vi "Handling AI param_Dll.vi"(4 "APCcode":i32[](array[numeric]), 5 "initialise":bool, 6 "AP":dbl[](array[numeric]), 7 "connect":bool[](array[boolean]), 8 "error in":errorcluster, 9 "input registers":u16[][](array[numeric]) format="%x", 10 "AI.AIP":refnum<data-value>, 11 "AI in":T1) -> (0 "error":errorcluster, 3 "AI out":T1)   [LabVIEW 2019, in "Inputs.lvlib"]
uses:
  Inputs.lvlib
  Ctl/AI short.ctl
  Ctl/Parameter State.ctl
  Timer Delay/Timers.lvlib
  src/libInputs.dll
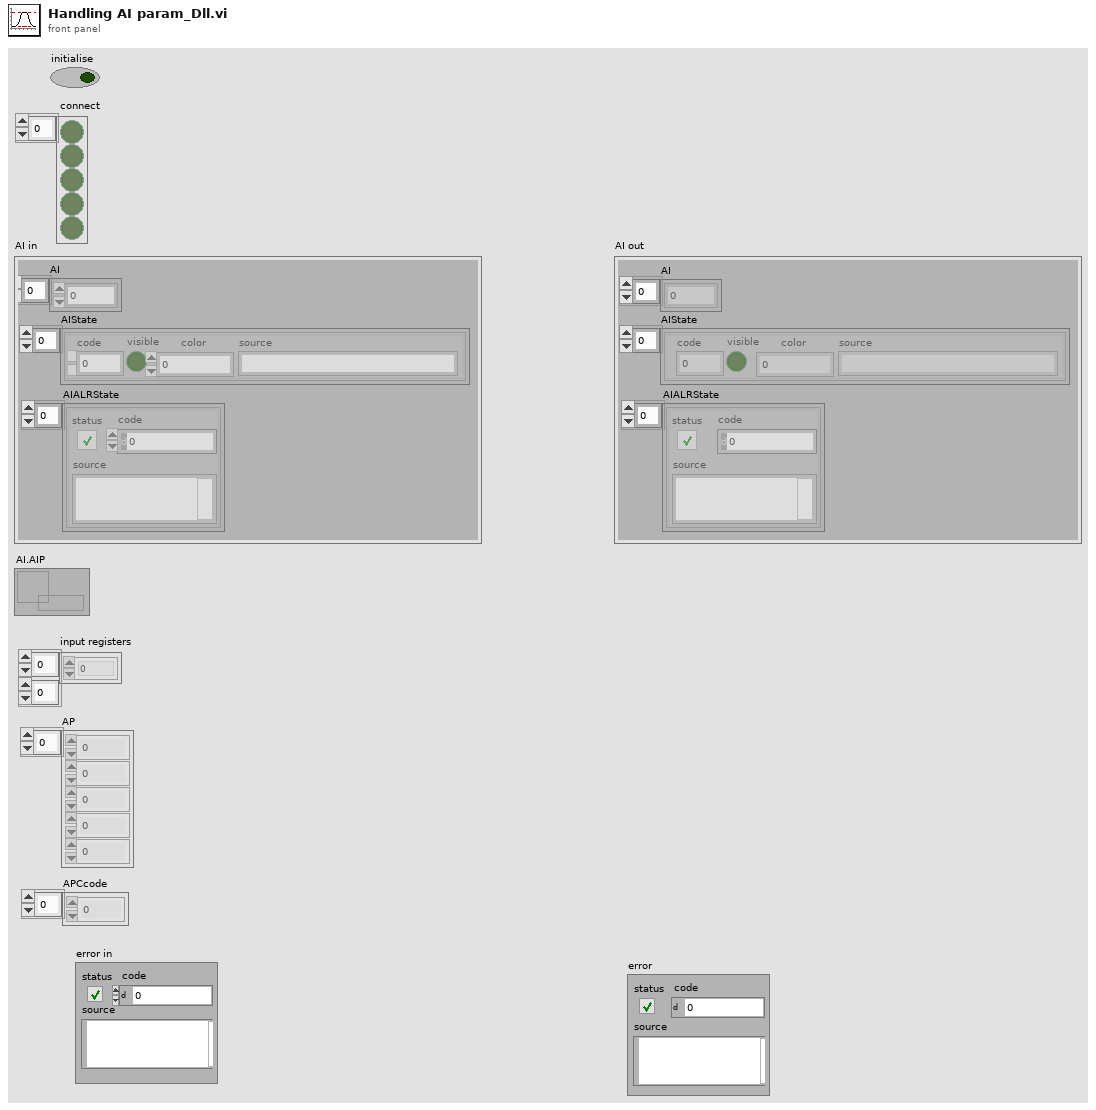
[diagram p1: front panel]
types:
  T1 = typedef "Inputs.lvlib/AI short.ctl" = cluster{"AI":dbl[], "AIState":T2[], "AIALRState":errorcluster[]}
  T2 = typedef "Inputs.lvlib/Parameter State.ctl" = cluster{"code":i32, "visible":bool, "color":u32, "source":string}
  T3 = cluster{"source":string, "color":u32, "visible":bool}[]
  T4 = cluster{"Filter PV_OUT":dbl, "Filter T":dbl, "Filter dT":dbl, "RS32 Q":u64}[]
  T5 = cluster{"Filter PV_OUT":dbl, "Filter T":dbl, "Filter dT":dbl, "RS32 Q":u64}
  T6 = cluster{"source":string, "color":u32, "visible":bool}
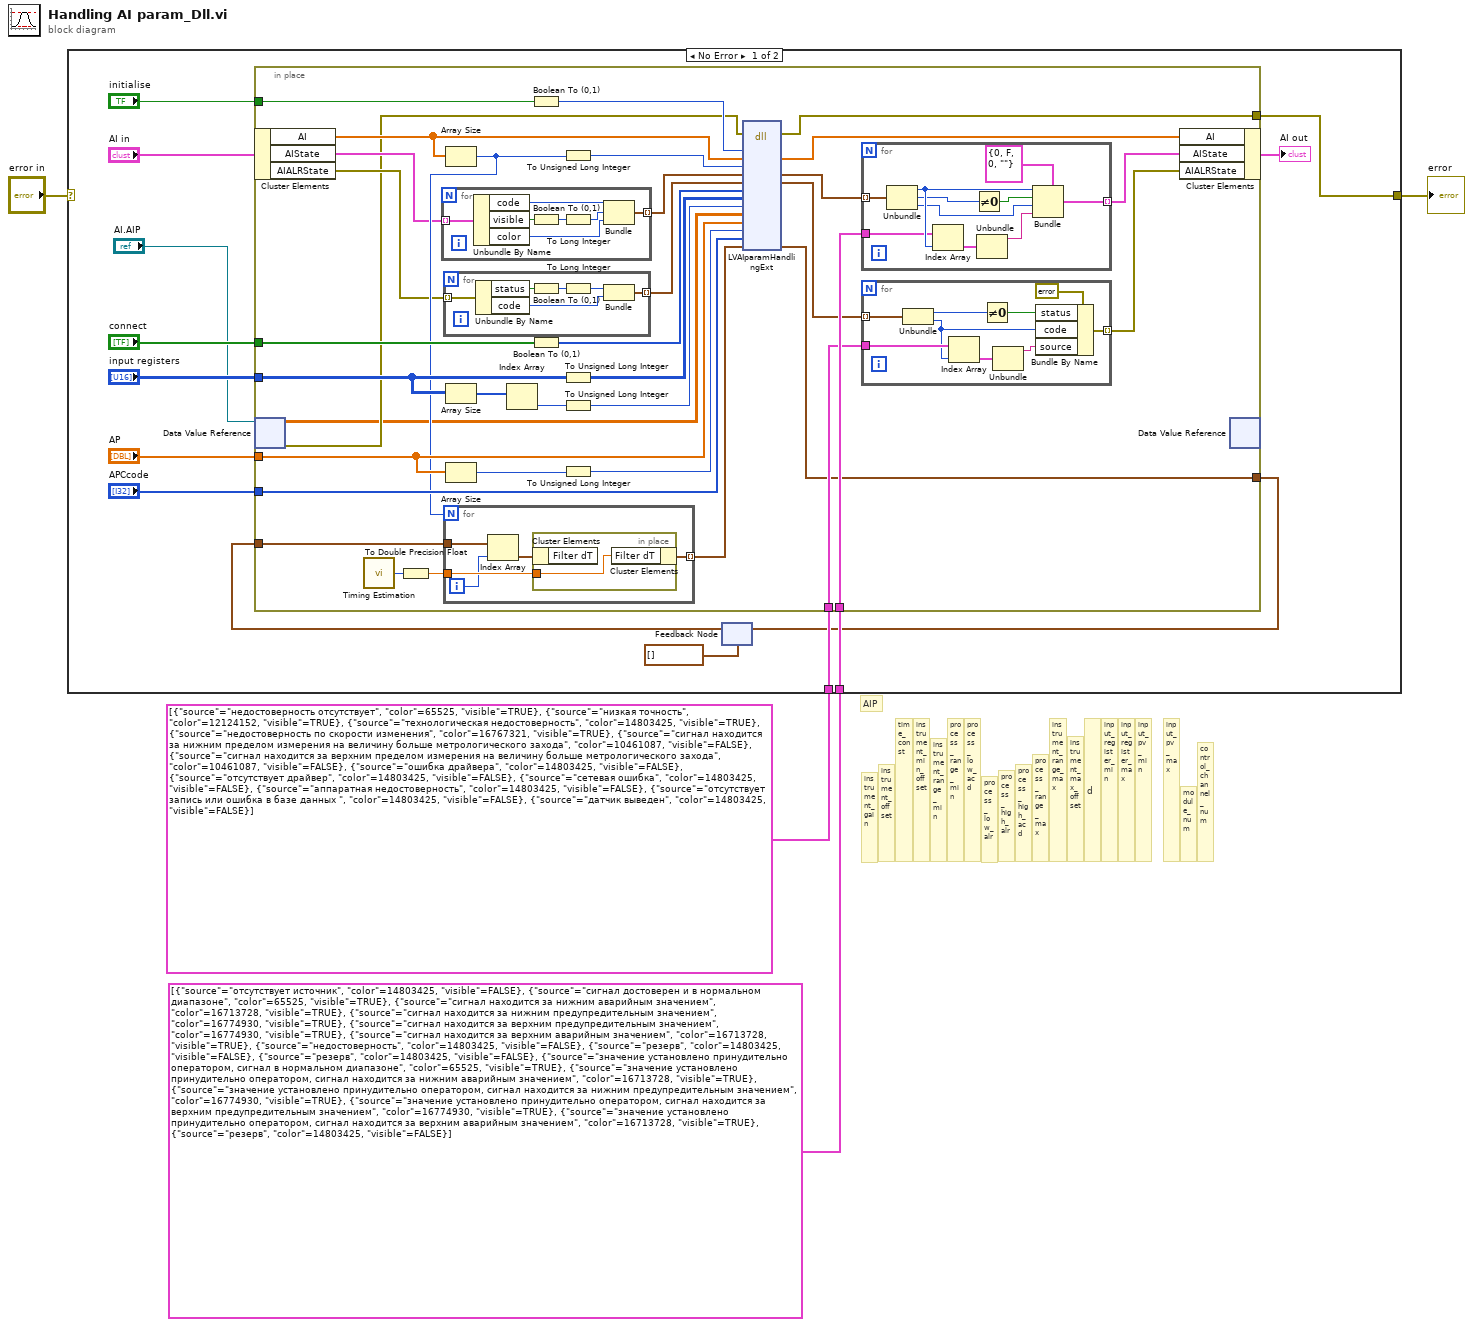
[diagram p0: block diagram]
diagram:
  # "AIP"
  # "control_channel_num"
  # "module_num"
  # "input_pv_max"
  # "input_pv_min"
  # "input_register_max"
  # "input_register_min"
  # "d"
  # "instrument_max_offset"
  # "instrument_range_max"
  # "process_range_max"
  # "process_high_acd"
  # "process_high_alr"
  # "process_low_alr"
  # "process_low_acd"
  # "process_range_min"
  # "instrument_range_min"
  # "instrument_min_offset"
  # "time_const"
  # "instrument_gain"
  # "instrument_offset"
  n1 = case shown="No Error" "error in" {
    selector: "error in" -> [_ w92]
    tunnel: T3 [{"source"="отсутствует источник", "color"=14803425, "visible"=FALSE}, {"source"="сигнал достоверен и в нормальном диапазоне", "color"=65525, "visible"=TRUE}, {"source"="сигнал находится за нижним аварийным значением", "color"=16713728, "visible"=TRUE}, {"source"="сигнал находится за нижним предупредительным значением", "color"=16774930, "visible"=TRUE}, {"source"="сигнал находится за верхним предупредительным значением", "color"=16774930, "visible"=TRUE}, {"source"="сигнал находится за верхним аварийным значением", "color"=16713728, "visible"=TRUE}, {"source"="недостоверность", "color"=14803425, "visible"=FALSE}, {"source"="резерв", "color"=14803425, "visible"=FALSE}, {"source"="резерв", "color"=14803425, "visible"=FALSE}, {"source"="значение установлено принудительно оператором, сигнал в нормальном диапазоне", "color"=65525, "visible"=TRUE}, {"source"="значение установлено принудительно оператором, сигнал находится за нижним аварийным значением", "color"=16713728, "visible"=TRUE}, {"source"="значение установлено принудительно оператором, сигнал находится за нижним предупредительным значением", "color"=16774930, "visible"=TRUE}, {"source"="значение установлено принудительно оператором, сигнал находится за верхним предупредительным значением", "color"=16774930, "visible"=TRUE}, {"source"="значение установлено принудительно оператором, сигнал находится за верхним аварийным значением", "color"=16713728, "visible"=TRUE}, {"source"="резерв", "color"=14803425, "visible"=FALSE}] -> [w16 _]
    tunnel: T3 [{"source"="недостоверность отсутствует", "color"=65525, "visible"=TRUE}, {"source"="низкая точность", "color"=12124152, "visible"=TRUE}, {"source"="технологическая недостоверность", "color"=14803425, "visible"=TRUE}, {"source"="недостоверность по скорости изменения", "color"=16767321, "visible"=TRUE}, {"source"="сигнал находится за нижним пределом измерения на величину больше метрологического захода", "color"=10461087, "visible"=FALSE}, {"source"="сигнал находится за верхним пределом измерения на величину больше метрологического захода", "color"=10461087, "visible"=FALSE}, {"source"="ошибка драйвера", "color"=14803425, "visible"=FALSE}, {"source"="отсутствует драйвер", "color"=14803425, "visible"=FALSE}, {"source"="сетевая ошибка", "color"=14803425, "visible"=FALSE}, {"source"="аппаратная недостоверность", "color"=14803425, "visible"=FALSE}, {"source"="отсутствует запись или ошибка в базе данных ", "color"=14803425, "visible"=FALSE}, {"source"="датчик выведен", "color"=14803425, "visible"=FALSE}] -> [w15 _]
    tunnel: [w8 w92] -> w2
    frame No Error {
      n2 = feedback #1(T4 []) -> (w10:T4)
      n3 = in-place {
        in-place-border: "initialise" -> [w53]
        in-place-border: "connect" -> [w52]
        in-place-border: w16 -> [w51]
        in-place-border: w15 -> [w50]
        in-place-border: "APCcode" -> [w49]
        in-place-border: "AP" -> [w48]
        in-place-border: "input registers" -> [w47]
        in-place-border: [w44] -> w11
        in-place-border: w10 -> [w43]
        in-place-border: [w27] -> w8
        n4 = in-place-cluster #2("AI in") -> ("AI"=w26:dbl[], "AIState"=w25:T2[], "AIALRState"=w24:errorcluster[])
        n5 = in-place-dvr #3("AI.AIP") -> (w19:dbl[][], w20:errorcluster)
        n6 = call "Timing Estimation.vi"() -> ("dt (ms) out"=w46:u32)  [unwired: 9 in]
        n7 = To Double Precision Float(number=w46) -> (double precision float=w45:dbl)
        n8 = for {
          tunnel: w25 -> [w66] mode=indexing
          tunnel: [w65] -> w37 mode=indexing
          n9 = Unbundle By Name(w66) -> ("code"=w64:i32, "visible"=w62:bool, "color"=w63:u32)
          n10 = Boolean To (0,1)(Boolean=w62) -> (0, 1=w61:i16)
          n11 = To Long Integer(number=w61) -> (32bit integer=w60:i32)
          n12 = Bundle("code"=w64, w60, "color"=w63) -> (w65:cluster{"code":i32, i32, "color":u32})  [unwired: 1 in]
        }
        n13 = for {
          tunnel: w24 -> [w72] mode=indexing
          tunnel: [w71] -> w36 mode=indexing
          n14 = Unbundle By Name(w72) -> ("status"=w69:bool, "code"=w70:i32)
          n15 = Boolean To (0,1)(Boolean=w69) -> (0, 1=w68:i16)
          n16 = To Long Integer(number=w68) -> (32bit integer=w67:i32)
          n17 = Bundle(w67, "code"=w70) -> (w71:cluster{i32, "code":i32})  [unwired: 1 in]
        }
        n18 = Array Size(array=w26) -> (size(s)=w28:i32)
        n19 = for {
          N: w28 -> [_]
          tunnel: w45 -> [w57]
          tunnel: w43 -> [w56]
          tunnel: [w58] -> w29 mode=indexing
          i -> [w54]
          n20 = Index Array(array=w56, index=w54) -> (element=w55:T5)
          n21 = in-place {
            in-place-border: w57 -> [w59]
            n22 = in-place-cluster #4(w55) -> ()  [unwired: 1 out]
            n23 = in-place-cluster #4("Filter dT"=w59) -> (w58:T5)
          }
        }
        n24 = Array Size(array=w47) -> (size(s)=w41:i32[])
        n25 = Array Size(array=w48) -> (size(s)=w40:i32)
        n26 = Index Array(array=w41) -> (element=w42:i32)  [unwired: 1 in]
        n27 = Boolean To (0,1)(Boolean=w53) -> (0, 1=w39:i16)
        n28 = Boolean To (0,1)(Boolean=w52) -> (0, 1=w32:i16[])
        n29 = To Unsigned Long Integer(number=w28) -> (unsigned 32bit integer=w38:u32)
        n30 = To Unsigned Long Integer(number=w47) -> (unsigned 32bit integer=w30:u32[][])
        n31 = To Unsigned Long Integer(number=w42) -> (unsigned 32bit integer=w31:u32)
        n32 = To Unsigned Long Integer(number=w40) -> (unsigned 32bit integer=w33:u32)
        n33 = dll-call lib="D:/my_projects/projects/Algorithms/Labview/19/Inputs/src/libInputs.dll" fn="LVAIparamHandlingExt"(error in=w20, "initialise"=w39, "AI"=w26, "AISize"=w38, "AIState"=w37, "AIAlrState"=w36, "connect"=w32, "InputRegisters"=w30, "InputRegistersSize"=w31, "AIParametersTable"=w19, "AP"=w48, "APSize"=w33, "APcode"=w49, "HAIPReg"=w29) -> (error out=w27:errorcluster, "AI"=w23:dbl[], "AIState"=w35:cluster{"code":i32, i32, "color":u32}[], "AIAlrState"=w34:cluster{i32, "code":i32}[], "HAIPReg"=w44:T4)  [unwired: 12 in, 1 out]
        n34 = for {
          tunnel: w35 -> [w82] mode=indexing
          tunnel: [w81] -> w22 mode=indexing
          tunnel: w51 -> [w79]
          n35 = Unbundle(w82) -> ("code"=w80:i32, w77:i32, "color"=w74:u32)
          n36 = Index Array(array=w79, index=w80) -> (element=w78:T6)
          n37 = Not Equal To 0?(x=w77) -> (x != 0?=w76:bool)
          n38 = Unbundle(w78) -> ("source"=w73:string)  [unwired: 2 out]
          n39 = Bundle(cluster=T2 {"code"=0, "visible"=FALSE, "color"=0, "source"=""} ("STATE"), "code"=w80, "visible"=w76, "color"=w74, "source"=w73) -> (w81:T2)
        }
        n40 = for {
          tunnel: w34 -> [w91] mode=indexing
          tunnel: [w90] -> w21 mode=indexing
          tunnel: w50 -> [w88]
          n41 = Unbundle(w91) -> (w85:i32, "code"=w86:i32)
          n42 = Index Array(array=w88, index=w86) -> (element=w89:T6)
          n43 = Not Equal To 0?(x=w85) -> (x != 0?=w84:bool)
          n44 = Unbundle(w89) -> ("source"=w87:string)  [unwired: 2 out]
          n45 = Bundle By Name(cluster=errorcluster {"status"=FALSE, "code"=0, "source"=""} ("ALRSTATE"), "status"=w84, "code"=w86, "source"=w87) -> (w90:errorcluster)
        }
        n46 = in-place-cluster #2("AI"=w23, "AIState"=w22, "AIALRState"=w21) -> (→"AI out":T1)
        n47 = in-place-dvr #3() -> ()  [unwired: 1 in, 2 out]
      }
      n48 = feedback-in #1(w11) -> ()
    }
    frame Error {
    }
  }
  "error" <- w2
